vi "AssertTrue.vi"(8 "error in (no error)":errorcluster, 10 "Message":string, 11 "Value":bool) -> (0 "error out":errorcluster)   [LabVIEW 2013]
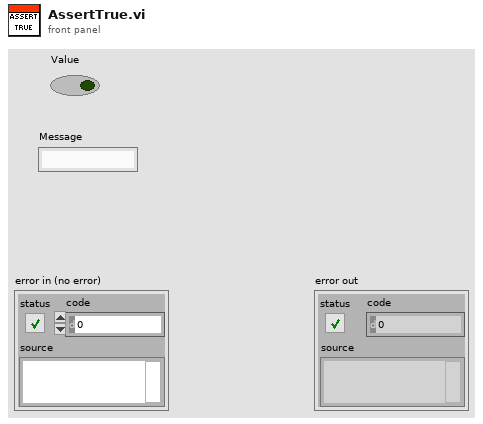
[diagram p1: front panel]
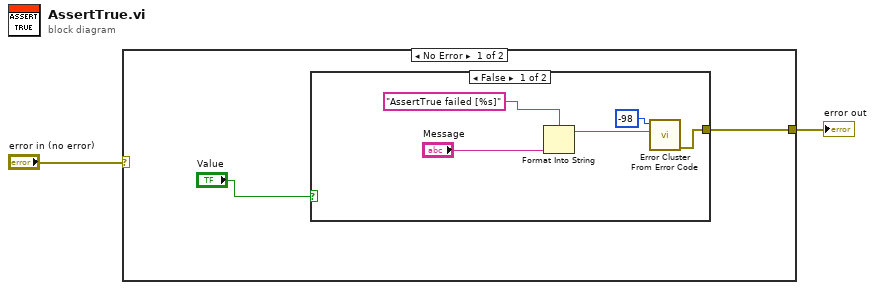
[diagram p0: block diagram]
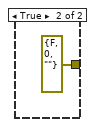
[diagram p2: hidden frame]
diagram:
  n1 = case shown="No Error" "error in (no error)" {
    selector: "error in (no error)" -> [_ w11]
    tunnel: [w4 w11] -> w1
    frame No Error {
      n2 = case shown="False" "Value" {
        tunnel: [w6 errorcluster {"status"=FALSE, "code"=0, "source"=""} ("error out")] -> w4
        frame False {
          n3 = Format Into String(format string="AssertTrue failed [%s]", "Message") -> (resulting string=w7:string)  [unwired: 2 in, 1 out]
          n4 = call <vilib>:"Error Cluster From Error Code.vi"("error message (\"\")"=w7, "error code (0)"=-98) -> ("error out"=w6:errorcluster)  [unwired: 7 in]
        }
        frame True {
        }
      }
    }
    frame Error {
    }
  }
  "error out" <- w1
